vi "enqueueEncoder.vi"(8 "error in (no error)":errorcluster, 11 "String":string) -> (0 "error out":errorcluster)   [LabVIEW 2017, in "externalAquisition.lvlib"]
uses:
  externalAquisition.lvlib
  TypeDefs/QueueCommands.ctl
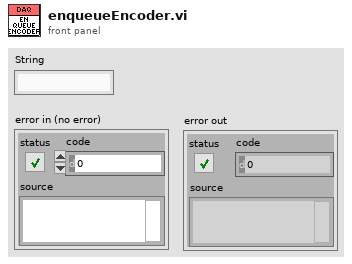
[diagram p1: front panel]
types:
  T1 = typedef "externalAquisition.lvlib/QueueCommands.ctl" = enum16{"get", "set"}
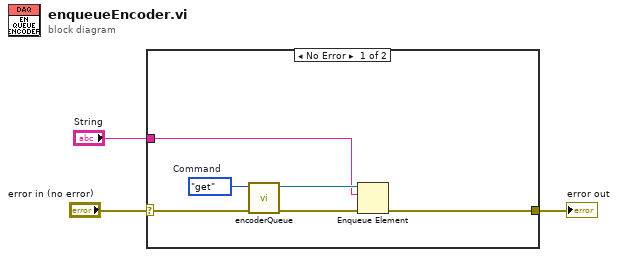
[diagram p0: block diagram]
diagram:
  n1 = case shown="No Error" "error in (no error)" {
    selector: "error in (no error)" -> [w9 w10]
    tunnel: [w5 w10] -> w2
    tunnel: "String" -> [w4 _]
    frame No Error {
      w8 = QueueCommands."get"  # Command
      n2 = call "encoderQueue.vi"("error in (no error)"=w9, "Command"=w8) -> ("error out"=w6:errorcluster, "queue out"=w7:refnum<queue>)  [unwired: 8 in]
      n3 = Enqueue Element(queue=w7, element=w4, error in (no error)=w6) -> (error out=w5:errorcluster)  [unwired: 1 in, 2 out]
    }
    frame Error {
    }
  }
  "error out" <- w2
